vi "Setlimit.vi"(8 "error in (no error)":errorcluster, 9 "Current":dbl, 10 "Voltage":dbl, 11 "B&K Precision 9120 series in":refnum<class "B&K Precision 9120 series.lvclass">) -> (0 "error out":errorcluster, 1 "Current read":dbl, 2 "Voltage read":dbl, 3 "B&K Precision 9120 series out":refnum<class "B&K Precision 9120 series.lvclass">)   [LabVIEW 2014, in "B&K Precision 9120 series.lvclass"]
uses:
  B&K Precision 9120 series.lvclass
  B&K Precision 9120 series.lvclass/B&K Precision 9120 series.ctl
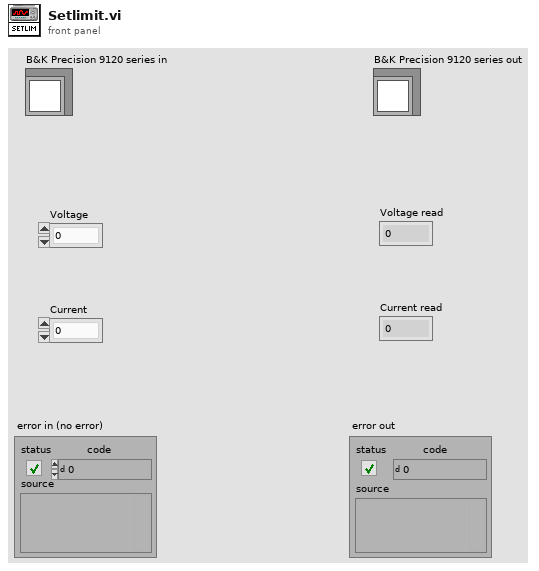
[diagram p1: front panel]
types:
  T1 = typedef "B&K Precision 9120 series.lvclass/Serial_Config.ctl" = cluster{"Baud":u32, "Flow Ctl":u16, "COM port":refnum<visa-resource-name>, "Parity":u16}
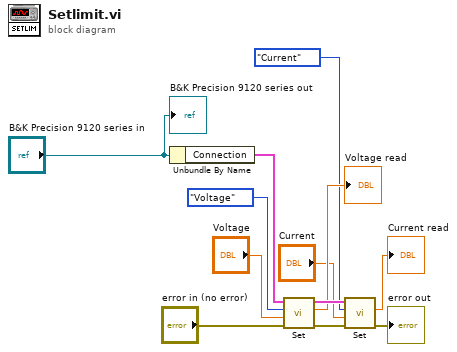
[diagram p0: block diagram]
diagram:
  n1 = Unbundle By Name("B&K Precision 9120 series in") -> ("Connection"=w11:T1)
  n2 = call "Set.vi"("Connection in"=w11, "Variable"=enum16{"Voltage", "Current"}."Voltage", "Value"="Voltage", "error in (no error)"="error in (no error)") -> ("Connection out"=w10:T1, "Actual Value"=→"Voltage read":dbl, "error out"=w6:errorcluster)  [unwired: 4 in]
  n3 = call "Set.vi"("Connection in"=w10, "Variable"=enum16{"Voltage", "Current"}."Current", "Value"="Current", "error in (no error)"=w6) -> ("Actual Value"=→"Current read":dbl, "error out"=→"error out":errorcluster)  [unwired: 4 in, 1 out]
  "B&K Precision 9120 series out" <- "B&K Precision 9120 series in"
